vi "Vector_Plotting.vi"(1 "Template Filename":path, 2 "Data":string[][](array[string]), 3 "Channel Names":string[](array[string])) -> ()   [LabVIEW 2011]
uses:
  Data_File_Type.ctl
  Controls/Group_Binning.ctl
  Globals/Constants_global.vi
panel:
  in  "Plot scalar Values":bool
  in  "V":u16(ring) items=["FF X", "FF Y", "FF Z", "Ch 1 Mean FF (C)", "Ch 1 Variance FF (C)", "X Source", "Y Source", "Z Source", "Ch 1 Bkgnd FF (C)", "Ch 1 Bkgnd Variance FF (C)", "Seconds since 1st Jan", "FF (C) Calibration Filename", "FF (C) Calibration Drift", "EnFlo_Tunnel FFID Temp", "Date of Measurement", "Time Measurement Commenced", "FF (C) Standard Error in Mean", "File", "Ch 1 Mean FF (C) Max Lat", "Ch 1 Mean FF (C) Sig Y", "Ch 1 Mean FF (C) Yo", "EnFlo_Tunnel Obstacle/ Building"]
  in  "U":u16(ring) items=["FF X", "FF Y", "FF Z", "Ch 1 Mean FF (C)", "Ch 1 Variance FF (C)", "X Source", "Y Source", "Z Source", "Ch 1 Bkgnd FF (C)", "Ch 1 Bkgnd Variance FF (C)", "Seconds since 1st Jan", "FF (C) Calibration Filename", "FF (C) Calibration Drift", "EnFlo_Tunnel FFID Temp", "Date of Measurement", "Time Measurement Commenced", "FF (C) Standard Error in Mean", "File", "Ch 1 Mean FF (C) Max Lat", "Ch 1 Mean FF (C) Sig Y", "Ch 1 Mean FF (C) Yo", "EnFlo_Tunnel Obstacle/ Building"]
  in  "Y Axis":u16(ring) items=["FF X", "FF Y", "FF Z", "Ch 1 Mean FF (C)", "Ch 1 Variance FF (C)", "X Source", "Y Source", "Z Source", "Ch 1 Bkgnd FF (C)", "Ch 1 Bkgnd Variance FF (C)", "Seconds since 1st Jan", "FF (C) Calibration Filename", "FF (C) Calibration Drift", "EnFlo_Tunnel FFID Temp", "Date of Measurement", "Time Measurement Commenced", "FF (C) Standard Error in Mean", "File", "Ch 1 Mean FF (C) Max Lat", "Ch 1 Mean FF (C) Sig Y", "Ch 1 Mean FF (C) Yo", "EnFlo_Tunnel Obstacle/ Building"]
  in  "X Axis":u16(ring) items=["FF X", "FF Y", "FF Z", "Ch 1 Mean FF (C)", "Ch 1 Variance FF (C)", "X Source", "Y Source", "Z Source", "Ch 1 Bkgnd FF (C)", "Ch 1 Bkgnd Variance FF (C)", "Seconds since 1st Jan", "FF (C) Calibration Filename", "FF (C) Calibration Drift", "EnFlo_Tunnel FFID Temp", "Date of Measurement", "Time Measurement Commenced", "FF (C) Standard Error in Mean", "File", "Ch 1 Mean FF (C) Max Lat", "Ch 1 Mean FF (C) Sig Y", "Ch 1 Mean FF (C) Yo", "EnFlo_Tunnel Obstacle/ Building"]
  in  "OK Button":bool
  in  "Row Selector":i32(listbox)=1
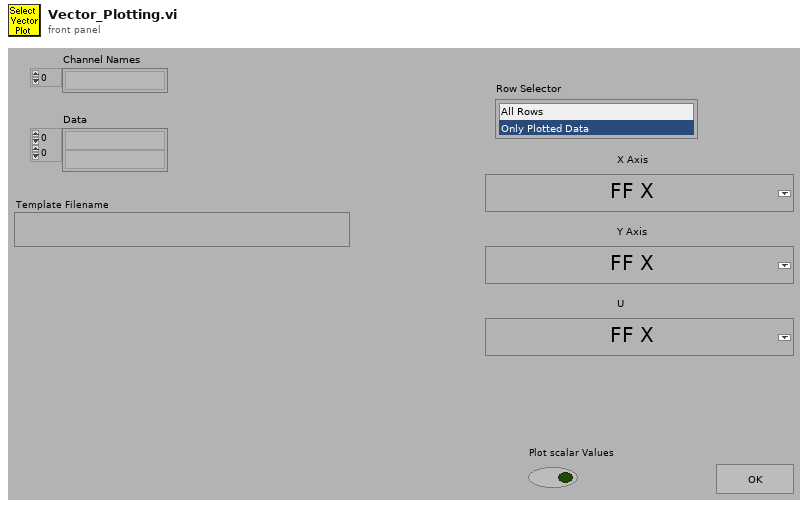
[diagram p1: front panel]
types:
  T1 = typedef "Data_File_Type.ctl" = enum16{"Read All File Types", "Results Files Only", "Raw Data Files Only", "Calibration Files Only", "Gas Desk Files Only", "Old Results Files Only", "Tabulated Data Files Only"}
  T2 = enum16{"Show only data summary", "Show data summary", "No data summary"}
  T3 = typedef "Group_Binning.ctl" = cluster{"Index":i32, "Tolerance":dbl, "Precision":string}
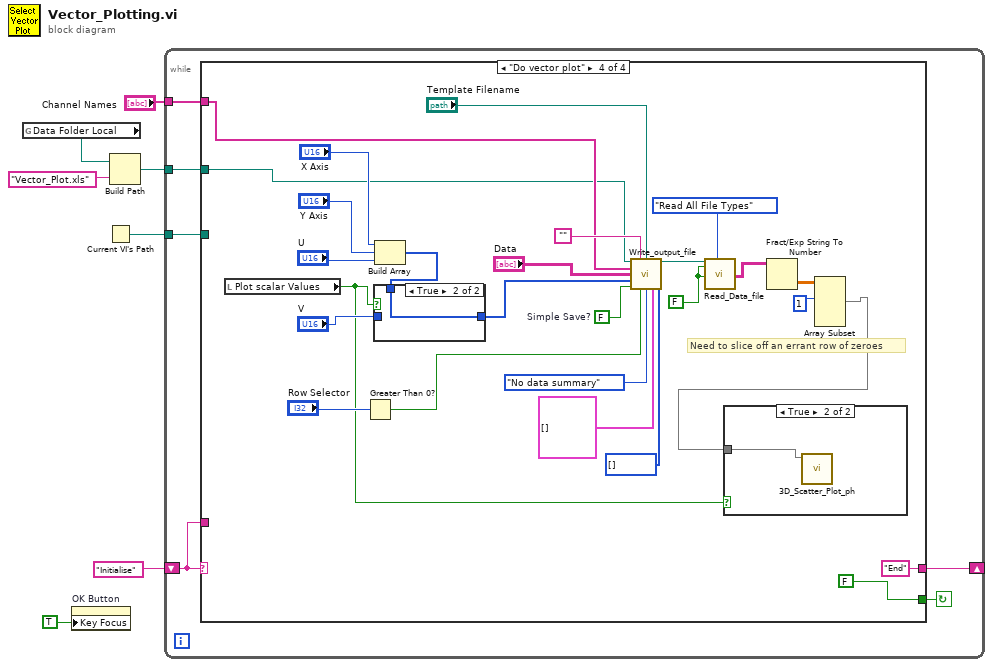
[diagram p0: block diagram]
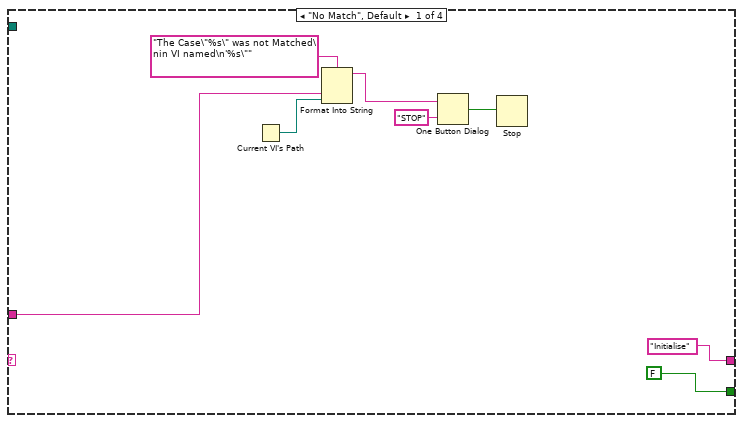
[diagram p2: hidden frame]
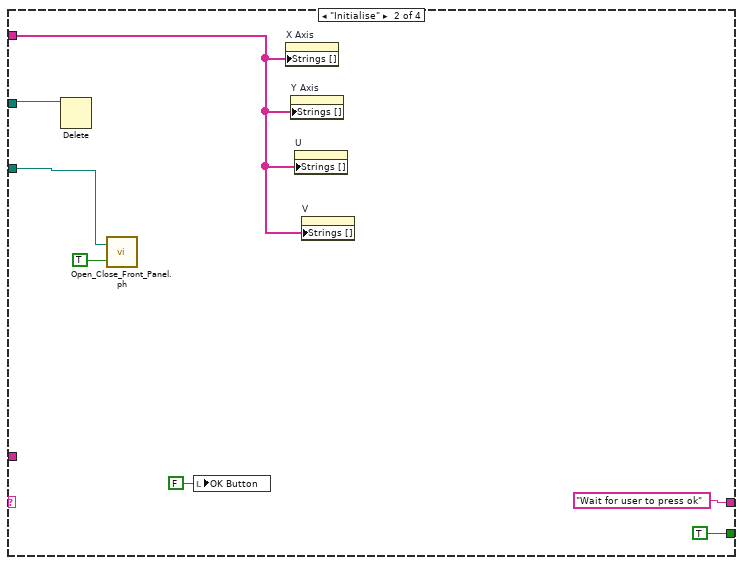
[diagram p3: hidden frame]
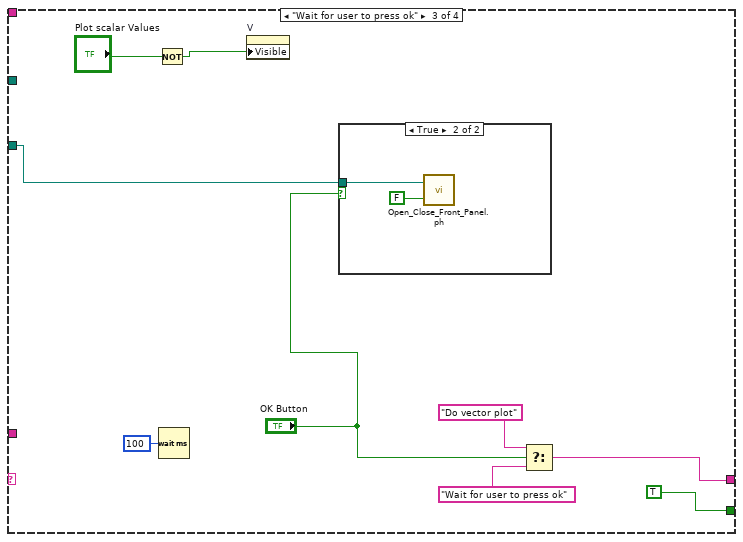
[diagram p4: hidden frame]
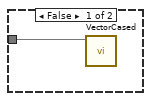
[diagram p6: hidden frame]
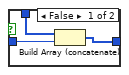
[diagram p7: hidden frame]
diagram:
  n1 = global read "Constants_global.vi" "Data Folder Local"() -> (w3:path)
  n2 = property on="OK Button" class="Bool (strict)"("Key Focus"=TRUE) -> ()  [unwired: 2 in, 2 out]
  n3 = Current VI's Path() -> (path=w6:path)
  n4 = Build Path(base path=w3, name or relative path="Vector_Plot.xls") -> (appended path=w1:path)
  n5 = while {
    shift-left: "Initialise" -> [w11]
    shift-right: [w12] -> _
    tunnel: w6 -> [w10]
    tunnel: "Channel Names" -> [w9]
    tunnel: w1 -> [w8]
    stop <- w13 continue-if-true
    n6 = case shown="\"Do vector plot\"" w11 {
      tunnel: [FALSE TRUE TRUE FALSE] -> w13
      tunnel: ["Initialise" "Wait for user to press ok" w36 "End" ("t")] -> w12
      tunnel: w11 -> [w16 _ _ _]
      tunnel: w10 -> [_ w26 w31 _]
      tunnel: w9 -> [_ w24 _ w49]
      tunnel: w8 -> [_ w22 _ w48]
      frame "No Match", Default {
        n7 = Current VI's Path() -> (path=w15:path)
        n8 = Format Into String(format string="The Case\"%s\" was not Matched\nin VI named\n'%s\"" ("Format String"), w16, w15) -> (resulting string=w19:string)  [unwired: 2 in, 1 out]
        n9 = One Button Dialog(message=w19, button name ("OK")="STOP") -> (true=w17:bool)
        n10 = Stop(stop? (T)=w17) -> ()
      }
      frame "Initialise" {
        n11 = Delete(path (use dialog)=w22) -> ()  [unwired: 1 in, 6 out]
        n12 = call "Open_Close_Front_Panel.ph.vi"("Front Panel Window:Open"=TRUE, "VI path"=w26) -> ()  [unwired: 2 out]
        n13 = local write "OK Button"(FALSE ("OK Button")) -> ()
        n14 = property on="X Axis" class="Ring (strict)"("Strings []"=w24) -> ()  [unwired: 2 in, 2 out]
        n15 = property on="Y Axis" class="Ring (strict)"("Strings []"=w24) -> ()  [unwired: 2 in, 2 out]
        n16 = property on="U" class="Ring (strict)"("Strings []"=w24) -> ()  [unwired: 2 in, 2 out]
        n17 = property on="V" class="Ring (strict)"("Strings []"=w24) -> ()  [unwired: 2 in, 2 out]
      }
      frame "Wait for user to press ok" {
        n18 = Not(x="Plot scalar Values") -> (.not. x?=w29:bool)
        n19 = Wait (ms)(milliseconds to wait=u32 100) -> ()  [unwired: 1 out]
        n20 = property on="V" class="Ring (strict)"("Visible"=w29) -> ()  [unwired: 2 in, 2 out]
        n21 = case shown="True" "OK Button" {
          tunnel: w31 -> [_ w38]
          frame False {
          }
          frame True {
            n22 = call "Open_Close_Front_Panel.ph.vi"("Front Panel Window:Open"=FALSE, "VI path"=w38) -> ()  [unwired: 2 out]
          }
        }
        n23 = Select(t="Do vector plot", s="OK Button", f="Wait for user to press ok") -> (s? t:f=w36:string)
      }
      frame "Do vector plot" {
        w52 = FALSE ("Read Channel Names only")
        w59 = FALSE  # Simple Save?
        # "Need to slice off an errant row of zeroes"
        n24 = local read "Plot scalar Values"() -> (w40:bool)
        n25 = Greater Than 0?(x="Row Selector") -> (x > 0?=w60:bool)
        n26 = Build Array("X Axis", "Y Axis", "U") -> (w43:u16[])
        n27 = case shown="True" w40 {
          tunnel: w43 -> [w71 w72]
          tunnel: "V" -> [w70 _]
          tunnel: [w69 w72] -> w41
          frame False {
            n28 = Build Array (concatenate)(w71, w70) -> (w69:u16[])
          }
          frame True {
          }
        }
        n29 = call "Write_output_file.vi"("Output filename"=w48, "Header"="", "Template Filename"="Template Filename", "Channel Names"=w49, "Data"="Data", "Desired Columns"=w41, "Simple Save?"=w59, "Save Plotted rows only?"=w60, "Summarise mode"=T2."No data summary", "Grouping info"=T3[] [], "Channels to Tabulate in header"=i32[] []) -> ("Output filename Out"=w53:path)  [unwired: 1 in, 3 out]
        n30 = call "Read_Data_file.vi"("Results file"=w53, "Read Channel Names only"=w52, "Add Extra Channels?"=w52, "Desired File Types"=Data_File_Type."Read All File Types") -> ("Channel Values Out"=w50:string[][])  [unwired: 1 in, 14 out]
        n31 = Fract/Exp String To Number(string=w50) -> (number=w46:dbl[][])  [unwired: 4 out]
        n32 = Array Subset(array=w46, index (row)=1 ("index")) -> (w45:dbl[][])  [unwired: 3 in]
        n33 = case shown="True" w40 {
          tunnel: w45 -> [w67 w68]
          frame False {
            n34 = call "VectorCased.vi"("XYUVArray"=w67) -> ()  [unwired: 11 out]
          }
          frame True {
            n35 = call "3D_Scatter_Plot_ph.vi"("XYUVArray"=w68) -> ()  [unwired: 11 in]
          }
        }
      }
    }
  }
